vi "3.vi"() -> ()   [LabVIEW 2017]
uses:
  <vilib>/measure/NI_MABase.lvlib
panel:
  out "Y":dbl[](array[numeric])
  in  "phase":dbl caption="相位" format="%.2p"
  in  "amplitude":dbl=1.0 caption="幅值" format="%0.2p"
  in  "frequency":dbl=10.0 caption="频率" format="%0.2p"
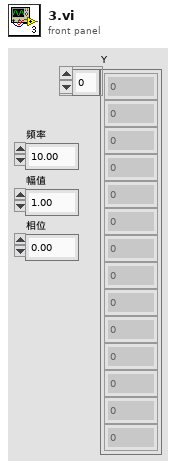
[diagram p1: front panel]
types:
  T1 = enum16{"open", "replace", "create", "open or create", "replace or create", "replace or create with confirmation"}
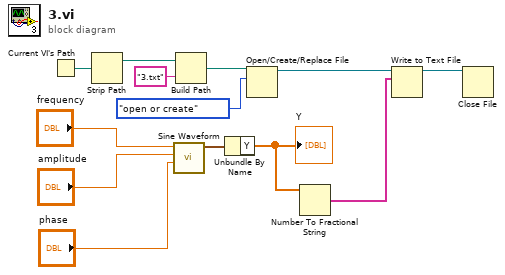
[diagram p0: block diagram]
diagram:
  n1 = Current VI's Path() -> (path=w13:path)
  n2 = Strip Path(path=w13) -> (stripped path=w12:path)  [unwired: 1 out]
  n3 = call <vilib>:"Sine Waveform.vi"("phase"="phase", "amplitude"="amplitude", "frequency"="frequency") -> ("signal out"=w7:waveform(dbl))  [unwired: 7 in, 1 out]
  n4 = Build Path(base path=w12, name or relative path="3.txt" ("名称或相对路径")) -> (appended path=w6:path)
  n5 = Unbundle By Name(w7) -> ("Y"=w3:dbl[])
  "Y" <- w3
  n6 = Open/Create/Replace File(file path (use dialog)=w6, operation (0:open)=T1."open or create" ("操作(0:open)")) -> (refnum out=w4:refnum<file>)  [unwired: 4 in, 2 out]
  n7 = Number To Fractional String(number=w3) -> (F-format string=w2:string[])  [unwired: 3 in]
  n8 = Write to Text File(file (use dialog)=w4, text=w2) -> (refnum out=w1:refnum<file>)  [unwired: 2 in, 2 out]
  n9 = Close File(refnum=w1) -> ()  [unwired: 1 in, 2 out]
